vi "Sleep Filter Wheel Stepper Motor.vi"(0 "Session Handle in":T1, 11 "error in (no error)":errorcluster) -> (4 "Session Handle out":T1, 6 "Success?":bool, 8 "Error Code":string, 15 "error out":errorcluster)   [LabVIEW 2015, in "PAS.lvclass"]
uses:
  PAS.lvclass
  Typedefs/Session Handle.ctl
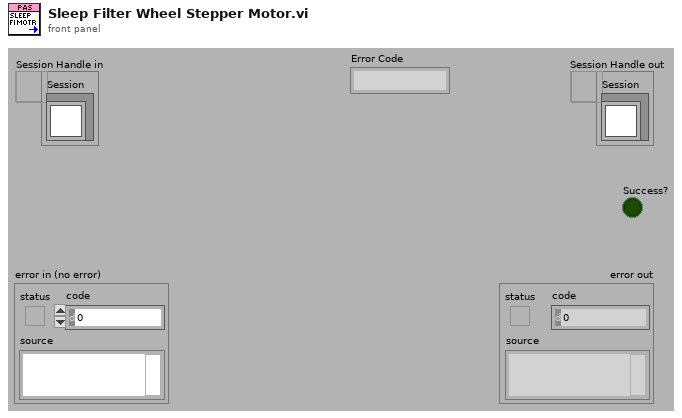
[diagram p1: front panel]
types:
  T1 = typedef "PAS.lvclass/Session Handle.ctl" = refnum<data-value>
  T2 = typedef "XNET Frame CAN.ctl" = cluster{"timestamp":timestamp, "payload":u8[], "identifier":u32, "type":T3, "extended?":bool, "echo?":bool}
  T3 = typedef "XNET Frame Type CAN.ctl" = u8
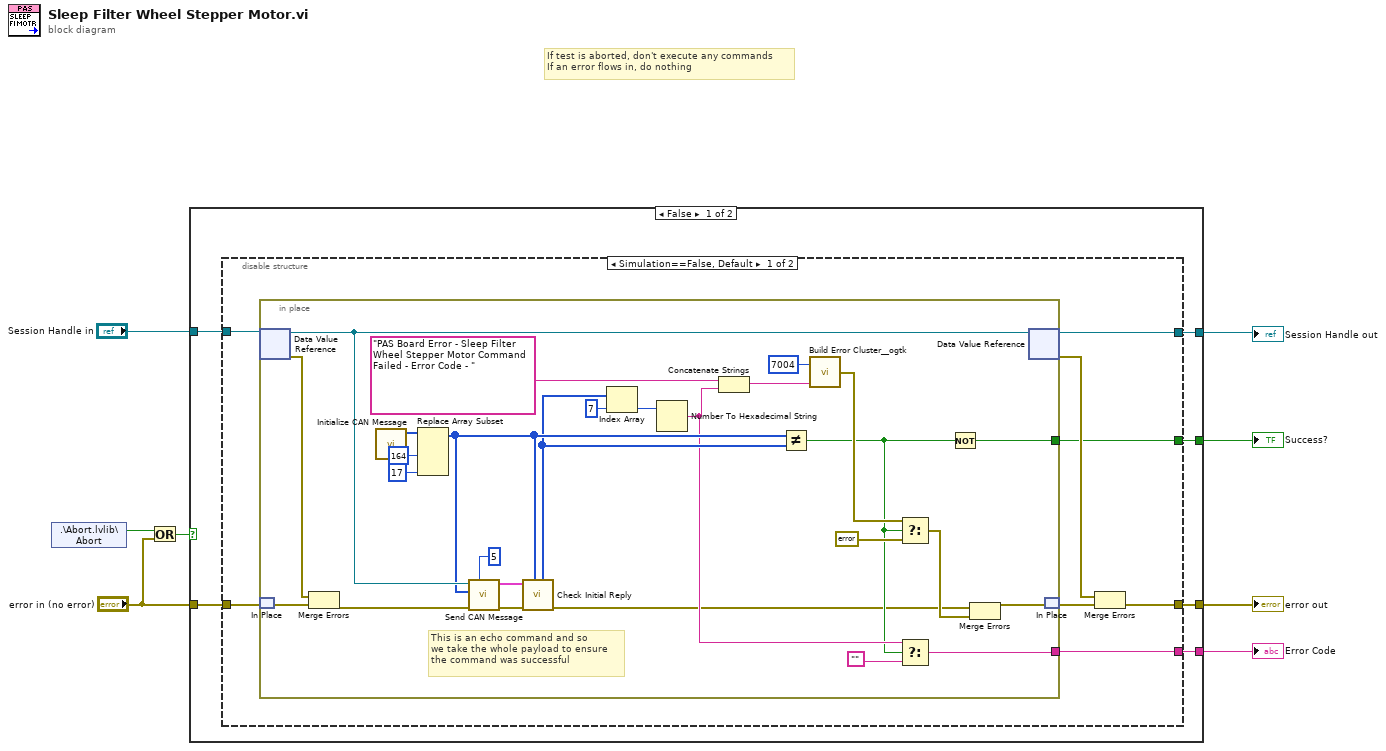
[diagram p0: block diagram]
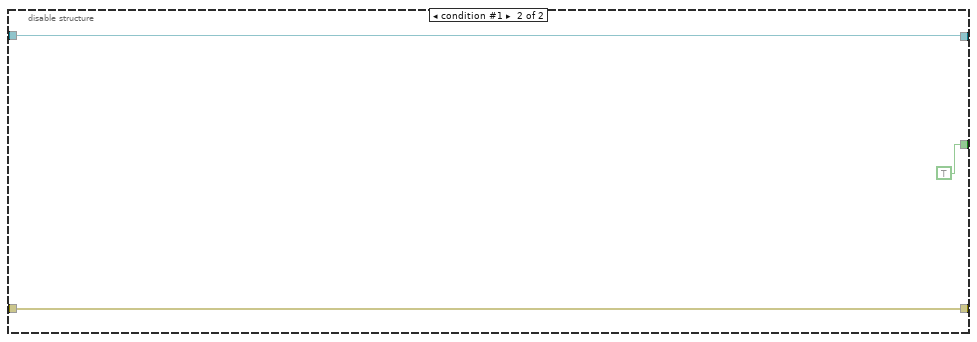
[diagram p2: hidden frame]
diagram:
  # "If test is aborted, don't execute any commands\nIf an error flows in, do nothing"
  n1 = shared-variable ".\\Abort.lvlib\\Abort"() -> (w5:bool)  [unwired: 1 in, 1 out]
  n2 = Or(x=w5, y="error in (no error)") -> (x .or. y?=w3:bool)
  n3 = case shown="False" w3 {
    tunnel: [w14 w54] -> w7
    tunnel: [w13 w53] -> w6
    tunnel: "Session Handle in" -> [w12 w54]
    tunnel: "error in (no error)" -> [w11 w53]
    tunnel: [w10 _] -> w2
    tunnel: [w9 _] -> w1
    frame False {
      n4 = disable-structure shown="Simulation==False, Default" {
        disable-tunnel: [w22 w52] -> w14
        disable-tunnel: [w19 w51] -> w13
        disable-tunnel: w12 -> [w18 w52]
        disable-tunnel: w11 -> [w17 w51]
        disable-tunnel: [w16 TRUE] -> w10
        disable-tunnel: [w15 _] -> w9
        frame condition #0 (active) {
          n5 = in-place {
            in-place-border: [w38] -> w16
            in-place-border: [w25] -> w15
            # "This is an echo command and so\nwe take the whole payload to ensure\nthe command was successful"
            n6 = in-place-dvr #1(w18) -> (w44:refnum<class "PAS.lvclass">, w47:errorcluster)
            n7 = in-place-match #2(w17) -> (w46:errorcluster)
            n8 = Merge Errors(w47, w46) -> (w45:errorcluster)
            n9 = call "Initialize CAN Message.vi"() -> ("Initial Payload"=w48:u8[])  [unwired: 11 in]
            n10 = Replace Array Subset(array=w48, new element #1=u8 164 ("new element/subarray"), new element #2=u8 17 ("new element/subarray")) -> (w37:u8[])  [unwired: 2 in]
            n11 = call "Send CAN Message.vi"("Number of Retries"=5, "error in (no error)"=w45, "payload"=w37, "Gas In"=w44) -> ("error out"=w24:errorcluster, "Reply"=w42:T2[])  [unwired: 5 in, 1 out]
            n12 = call "Check Initial Reply.vi"("Write Message"=w37, "error in (no error)"=w24, "Reply"=w42) -> ("error out"=w23:errorcluster, "Whole Payload"=w31:u8[])  [unwired: 5 in, 2 out]
            n13 = Index Array(array=w31, index=7) -> (element=w29:u8)
            n14 = Number To Hexadecimal String(2:w29) -> (0:w27:string)  [unwired: 1 in]
            n15 = Concatenate Strings("PAS Board Error - Sleep Filter Wheel Stepper Motor Command Failed - Error Code - " ("string"), w27) -> (w32:string)
            n16 = Not Equal?(x=w37, y=w31) -> (x != y?=w26:bool)
            n17 = call <userlib>:"Build Error Cluster__ogtk.vi"("String to Prepend to source (\"\")"=w32, "code"=7004) -> ("error out"=w40:errorcluster)
            n18 = Select(t=w40, s=w26, f=errorcluster {"status"=FALSE, "code"=0, "source"=""}) -> (s? t:f=w34:errorcluster)
            n19 = Select(t=w27, s=w26, f="") -> (s? t:f=w25:string)
            n20 = Not(x=w26) -> (.not. x?=w38:bool)
            n21 = Merge Errors(w23, w34) -> (w35:errorcluster)
            n22 = in-place-dvr #1(w44) -> (w22:T1, w20:errorcluster)
            n23 = in-place-match #2(w35) -> (w21:errorcluster)
          }
          n24 = Merge Errors(w20, w21) -> (w19:errorcluster)
        }
        frame condition #1 {
        }
      }
    }
    frame True {
    }
  }
  "Session Handle out" <- w7
  "error out" <- w6
  "Success?" <- w2
  "Error Code" <- w1
